vi "PartialClusterWithStrings.vi"(11 "Cluster":T2={"String To Append"="", "String"="", "Array 1"=["Has ", "Default ", "Values"], "Array 2"=["Has ", "More ", "Default ", "Values"], "String 2"="This is a default value"}) -> (3 "Cluster 2":T1)   [LabVIEW 2013]
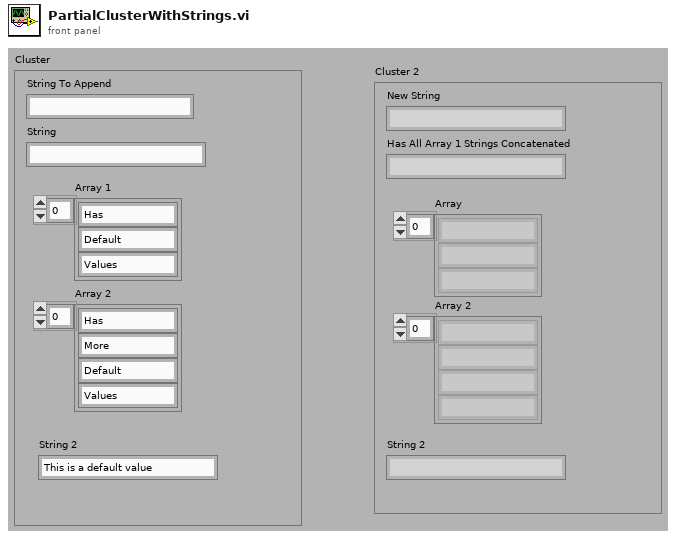
[diagram p1: front panel]
types:
  T1 = cluster{"New String":string, "Has All Array 1 Strings Concatenated":string, "Array":string[], "Array 2":string[], "String 2":string}
  T2 = cluster{"String To Append":string, "String":string, "Array 1":string[], "Array 2":string[], "String 2":string}
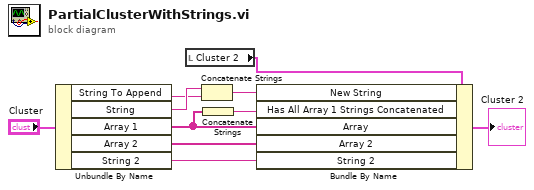
[diagram p0: block diagram]
diagram:
  n1 = Unbundle By Name("Cluster") -> ("String To Append"=w1:string, "String"=w2:string, "Array 1"=w5:string[], "Array 2"=w4:string[], "String 2"=w3:string)
  n2 = local read "Cluster 2"() -> (w8:T1)
  n3 = Concatenate Strings(w2, w1) -> (w7:string)
  n4 = Concatenate Strings(w5) -> (w6:string)
  n5 = Bundle By Name(cluster=w8, "New String"=w7, "Has All Array 1 Strings Concatenated"=w6, "Array"=w5, "Array 2"=w4, "String 2"=w3) -> (→"Cluster 2":T1)
